vi "Get ChildHwnd[].vi"(0 "LV MDI in":refnum<class "LV MDI.lvclass">, 11 "error in (no error)":errorcluster) -> (4 "LV MDI out":refnum<class "LV MDI.lvclass">, 6 "ChildHwnd[]":u32[](array[numeric]), 15 "error out":errorcluster)   [LabVIEW 2016, in "LV MDI.lvclass"]
doc: "Get all Child Window Hwnd."
uses:
  LV MDI.lvclass
  LV MDI.lvclass/LV MDI.ctl
  Document/Document.lvclass/Document.ctl
  Document/Document.lvclass
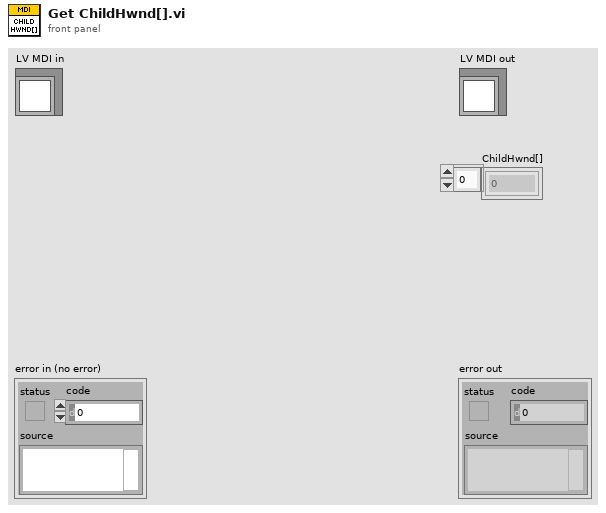
[diagram p1: front panel]
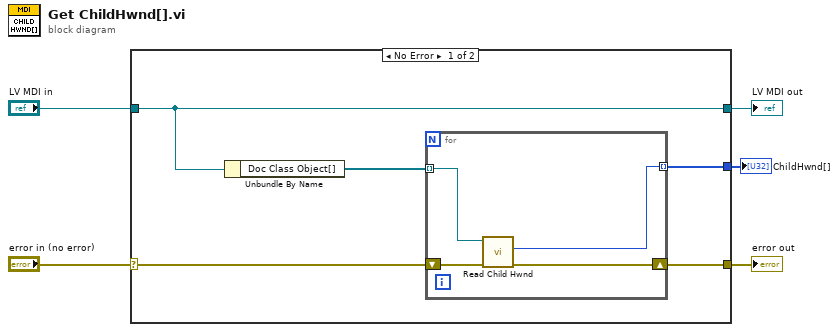
[diagram p0: block diagram]
diagram:
  n1 = case shown="No Error" "error in (no error)" {
    selector: "error in (no error)" -> [w9 w16]
    tunnel: [w8 w16] -> w4
    tunnel: [w10 w15] -> w2
    tunnel: "LV MDI in" -> [w10 w15]
    tunnel: [w6 _] -> w1
    frame No Error {
      n2 = Unbundle By Name(w10) -> ("Doc Class Object[]"=w7:refnum<class "Document.lvclass">[])
      n3 = for {
        shift-right: [w13] -> w8
        shift-left: w9 -> [w14]
        tunnel: w7 -> [w11] mode=indexing
        tunnel: [w12] -> w6 mode=indexing
        n4 = call "Read Child Hwnd.vi"("error in (no error)"=w14, "Document in"=w11) -> ("error out"=w13:errorcluster, "Child Hwnd"=w12:u32)  [unwired: 7 in, 1 out]
      }
    }
    frame Error {
    }
  }
  "error out" <- w4
  "LV MDI out" <- w2
  "ChildHwnd[]" <- w1
